vi "Main.vi"(7 "Actor":refnum<class "Actor.lvclass">) -> ()   [LabVIEW 2020, in "jettl.lvlib" / "Actor.lvclass"]
uses:
  Actor.lvclass
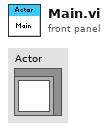
[diagram p1: front panel]
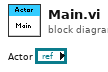
[diagram p0: block diagram]
diagram:
